vi "KE2000_CommandsGlobal.vi"() -> ()   [LabVIEW 2019, in "KE2000.lvclass"]
uses:
  KE2000.lvclass
panel:
  in  "Keithley 2000 GPIB Setup":T1={"Instrument name"="Keithley 2000", "Command \"Reset\""=":INIT:CONT 0;:ABOR;*CLS;*RST", "Command \"Initialise\""="%s;%s;:SENS:VOLT:DC:NPLC 10;:SENS:CURR:DC:NPLC 10", "Command \"Read Data\""=":READ?"}
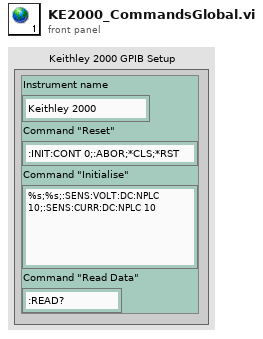
[diagram p1: front panel]
types:
  T1 = cluster{"Instrument name":string, "Command \"Reset\"":string, "Command \"Initialise\"":string, "Command \"Read Data\"":string}
diagram:
